vi "PiezoSetVoltage.vi"(8 "error in":errorcluster, 10 "data":dbl[](array[numeric]) format="%0.2f") -> (0 "error out":errorcluster)   [LabVIEW 2015]
uses:
  <vilib>/DAQmx/write.llb/DAQmx Write.vi
  <vilib>/DAQmx/write.llb/DAQmx Write (Analog 1D DBL NChan 1Samp).vi
  <vilib>/DAQmx/miscellaneous.llb/DAQmx Fill In Error Info.vi
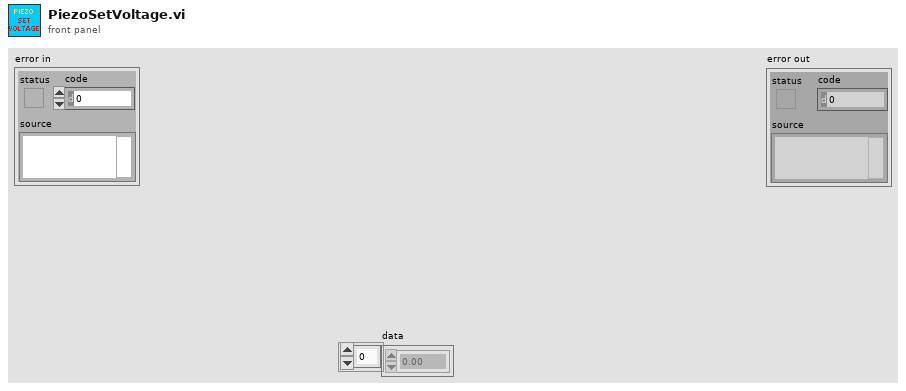
[diagram p1: front panel]
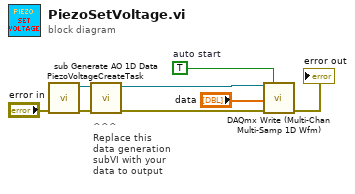
[diagram p0: block diagram]
diagram:
  w3 = TRUE  # auto start
  # "^^^\nReplace this\ndata generation\nsubVI with your\ndata to output"
  n1 = call "PiezoVoltageCreateTask.vi"("error in"="error in") -> ("error out"=w7:errorcluster, "task out"=w6:refnum<k21>)  [unwired: 9 in]
  n2 = call <vilib>:"sub Generate AO 1D Data.vi"("error in"=w7, "task in"=w6) -> ("error out"=w5:errorcluster, "task out"=w4:refnum<k21>)  [unwired: 7 in, 1 out]
  n3 = call-poly "DAQmx Write (Multi-Chan Multi-Samp 1D Wfm).vi"("task/channels in"=w4, "auto start"=w3, "data"="data", "error in"=w5) -> ("error out"=→"error out":errorcluster)  [unwired: 9 in, 2 out]
